vi "GPS通讯(子VI).vi"(8 "error in (no error)":errorcluster caption="错误输入（无错误）") -> ()   [LabVIEW 2016, in "环境动力监测库.lvlib" / "NMEA.lvlib"]
uses:
  NMEA.lvlib
  <vilib>/Plasmionique/MB Master/MB_Master/MB_Master.lvclass
  <vilib>/Plasmionique/MB Master/MB_Master_TCP/MB_Master_TCP.lvclass
  D:/Program Files (x86)/National Instruments/LabVIEW 2016/vi.lib/Plasmionique/MB Master/MB_Master/MB_Master.lvclass
  <vilib>/Instr/_visa.llb/VISA Configure Serial Port (Instr).vi
  <vilib>/Plasmionique/MB Master/MB Master.lvlib
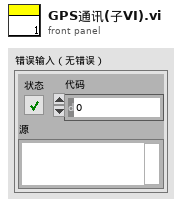
[diagram p1: front panel]
types:
  T1 = cluster{"定位状态":bool, "卫星数量":u16, "时间标识":timestamp, "纬度":dbl, "南北":string, "经度":dbl, "东西":string}
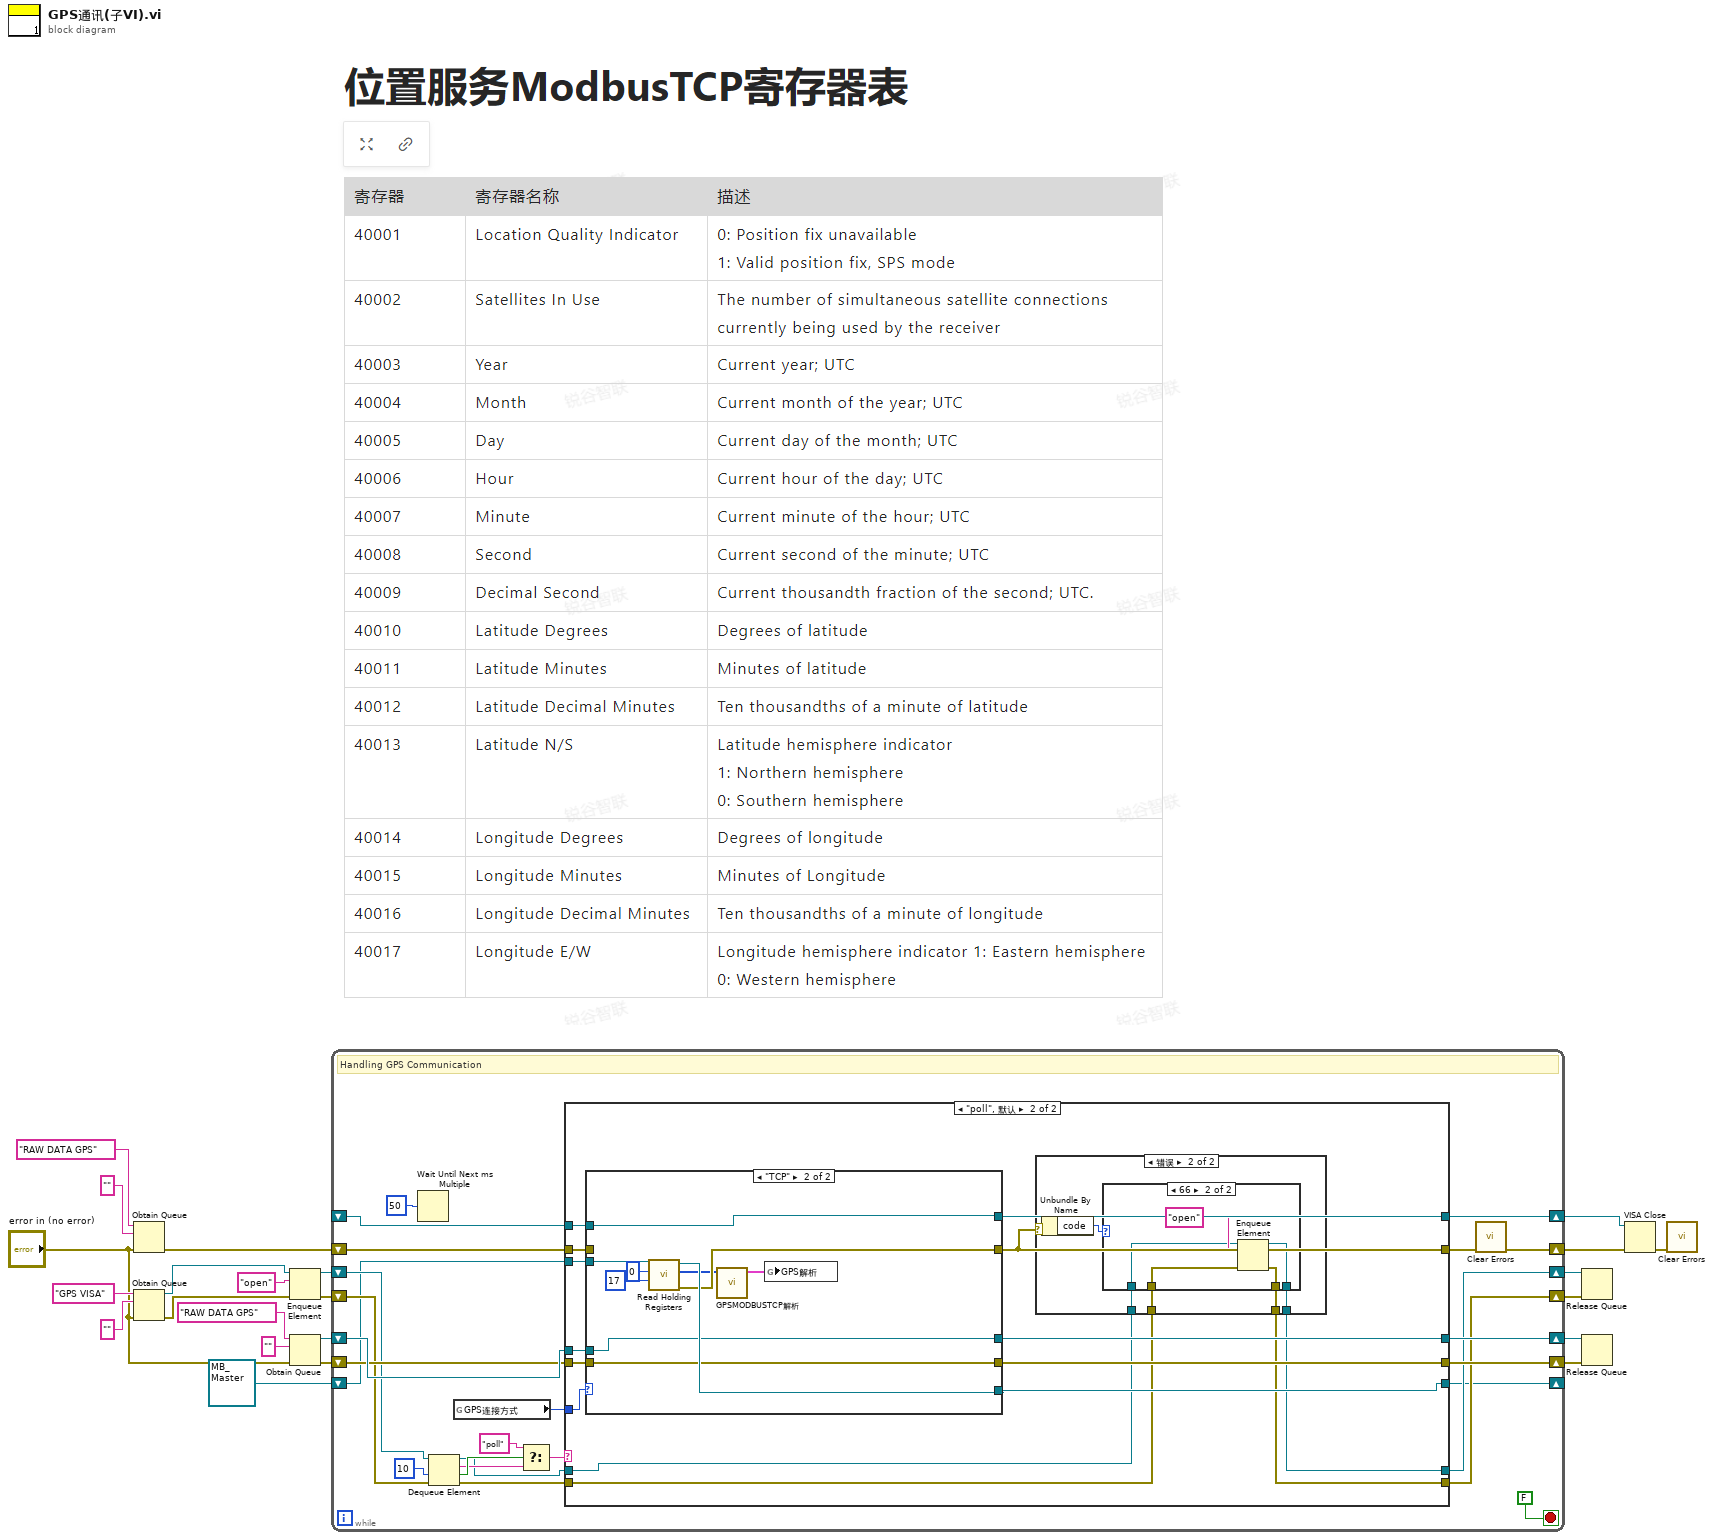
[diagram p0: block diagram]
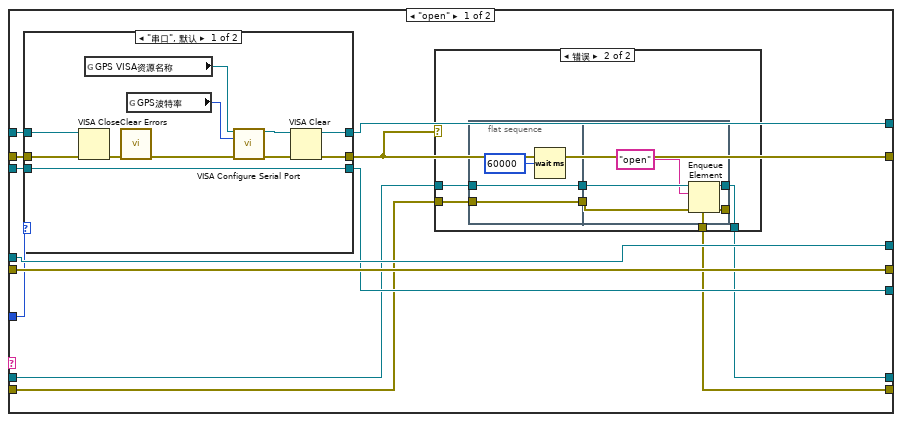
[diagram p2: hidden frame]
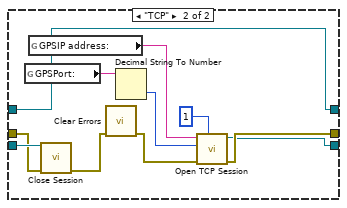
[diagram p4: hidden frame]
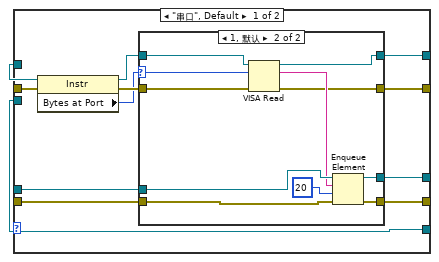
[diagram p7: hidden frame]
diagram:
  n1 = Obtain Queue(name (unnamed)="RAW DATA GPS" ("nom (aucun)"), element data type="" ("expression régulière"), error in (no error)="error in (no error)") -> (error out=w14:errorcluster)  [unwired: 2 in, 2 out]
  n2 = Obtain Queue(name (unnamed)="GPS VISA" ("名称（未命名）"), element data type="" ("名称（未命名）"), error in (no error)="error in (no error)") -> (queue out=w11:refnum<queue>, error out=w10:errorcluster)  [unwired: 2 in, 1 out]
  n3 = Enqueue Element(queue=w11, element="open" ("元素"), error in (no error)=w10) -> (queue out=w8:refnum<queue>, error out=w7:errorcluster)  [unwired: 1 in, 1 out]
  n4 = Obtain Queue(name (unnamed)="RAW DATA GPS" ("nom (aucun)"), element data type="" ("expression régulière"), error in (no error)="error in (no error)") -> (queue out=w4:refnum<queue>, error out=w3:errorcluster)  [unwired: 2 in, 1 out]
  n5 = while {
    shift-right: [w45] -> w18
    shift-left: w3 -> [w47]
    shift-right: [w44] -> w20
    shift-left: _ -> [w43]
    shift-right: [w46] -> w19
    shift-left: w4 -> [w48]
    shift-right: [w39] -> w21
    shift-left: w14 -> [w41]
    shift-right: [w29] -> w22
    shift-left: w7 -> [w37]
    shift-right: [w31] -> w23
    shift-left: w8 -> [w38]
    shift-right: [w25] -> _
    shift-left: refnum<class "MB_Master.lvclass"> refnum ("MB session in") -> [w24]
    stop <- FALSE stop-if-true
    # "Handling GPS Communication"
    n6 = Wait Until Next ms Multiple(millisecond multiple=u32 50 ("attente (ms)")) -> ()  [unwired: 1 out]
    n7 = Dequeue Element(queue=w38, timeout in ms (-1)=10 ("超时毫秒(-1)"), error in (no error)=w37) -> (queue out=w30:refnum<queue>, element=w33:string, timed out?=w35:bool, error out=w28:errorcluster)
    n8 = global read "断电保存全局变量.vi" "GPS连接方式"() -> (w26:enum16{"串口", "TCP"})
    n9 = Select(t="poll" ("名称（未命名）"), s=w35, f=w33) -> (s? t:f=w32:string)
    n10 = case shown="\"poll\", 默认" w32 {
      tunnel: w48 -> [w61 w114]
      tunnel: w47 -> [w60 w113]
      tunnel: [w61 w112] -> w46
      tunnel: [w60 w111] -> w45
      tunnel: [w57 w110] -> w44
      tunnel: w43 -> [w58 w109]
      tunnel: w41 -> [w59 w108]
      tunnel: [w53 w104] -> w40
      tunnel: [w50 w100] -> w31
      tunnel: w30 -> [w52 w103]
      tunnel: [w49 w101] -> w29
      tunnel: w28 -> [w51 w102]
      tunnel: w26 -> [w56 w107]
      tunnel: [w55 w105] -> w25
      tunnel: w24 -> [w54 w106]
      frame "open" {
        n11 = case shown="\"串口\", 默认" w56 {
          tunnel: w59 -> [w85 w91]
          tunnel: w58 -> [w84 w99]
          tunnel: [w81 w99] -> w57
          tunnel: [w79 w93] -> w53
          tunnel: [w78 w89] -> w55
          tunnel: w54 -> [w78 w92]
          frame "串口", Default {
            n12 = VISA Close(VISA resource name=w84, error in (no error)=w85) -> (error out=w83:errorcluster)
            n13 = global read "断电保存全局变量.vi" "GPS VISA资源名称"() -> (w87:refnum<visa-resource-name>)
            n14 = call <vilib>:"Clear Errors.vi"("error in (no error)"=w83) -> ("error out"=w82:errorcluster)  [unwired: 5 in, 1 out]
            n15 = global read "断电保存全局变量.vi" "GPS波特率"() -> (w88:u32)
            n16 = call-poly "VISA Configure Serial Port"("VISA resource name"=w87, "baud rate (9600)"=w88, "error in (no error)"=w82) -> ("VISA resource name out"=w86:refnum<visa-resource-name>, "error out"=w80:errorcluster)  [unwired: 11 in]
            n17 = VISA Clear(VISA resource name=w86, error in (no error)=w80) -> (VISA resource name out=w81:refnum<visa-resource-name>, error out=w79:errorcluster)
          }
          frame "TCP" {
            n18 = global read "断电保存全局变量.vi" "GPSPort:"() -> (w96:string)
            n19 = global read "断电保存全局变量.vi" "GPSIP address:"() -> (w97:string)
            n20 = call-dynamic "Close Session.vi"("error in (no error)"=w91, "MB session in"=w92) -> ("error out"=w90:errorcluster)  [unwired: 9 in]
            n21 = call <vilib>:"Clear Errors.vi"("error in (no error)"=w90) -> ("error out"=w94:errorcluster)  [unwired: 5 in, 1 out]
            n22 = Decimal String To Number(string=w96) -> (number=w95:i32)  [unwired: 2 in, 1 out]
            n23 = call <vilib>:"Open TCP Session.vi"("Slave ID (255)"=u8 1, "error in (no error)"=w94, "Port (502)"=w95, "IP Address"=w97) -> ("error out"=w93:errorcluster, "MB_TCP session"=w89:refnum<class "MB_Master_TCP.lvclass">)  [unwired: 6 in]
          }
        }
        n24 = case shown="错误" w53 {
          tunnel: w52 -> [w63 w69]
          tunnel: w51 -> [w62 w68]
          tunnel: [w63 w67] -> w50
          tunnel: [w62 w66] -> w49
          frame No Error {
          }
          frame Error {
            n25 = flat-sequence {
              tunnel: w68 -> [w71]
              tunnel: w69 -> [w72]
              tunnel: [w72] -> w65
              tunnel: [w71] -> w64
              tunnel: [w74] -> w67
              tunnel: [w73] -> w66
              tunnel: w65 -> [w77]
              tunnel: w64 -> [w76]
              frame #0 {
                n26 = Wait (ms)(milliseconds to wait=u32 60000 ("等待时间（毫秒）")) -> ()  [unwired: 1 out]
              }
              frame #1 {
                n27 = Enqueue Element(queue=w77, element="open" ("名称（未命名）"), error in (no error)=w76) -> (queue out=w74:refnum<queue>, error out=w73:errorcluster)  [unwired: 1 in, 1 out]
              }
            }
          }
        }
      }
      frame "poll", Default {
        n28 = case shown="\"TCP\"" w107 {
          tunnel: w114 -> [w141 w160]
          tunnel: w113 -> [w140 w159]
          tunnel: [w139 w160] -> w112
          tunnel: [w138 w159] -> w111
          tunnel: [w137 w166] -> w110
          tunnel: w109 -> [w136 w166]
          tunnel: w108 -> [w135 _]
          tunnel: [w134 w161] -> w104
          tunnel: w106 -> [w130 w165]
          tunnel: [w130 w162] -> w105
          frame "串口", Default {
            n29 = property class="Instr"(reference=w136, error in=w135) -> (reference out=w133:refnum<visa-resource-name>, error out=w132:errorcluster, "Bytes at Port"=w131:u32)
            n30 = case shown="1, 默认" w131 {
              selector: w131 -> [_ w147]
              tunnel: w141 -> [w142 w156]
              tunnel: w140 -> [w143 w155]
              tunnel: [w142 w154] -> w139
              tunnel: [w143 w153] -> w138
              tunnel: [w144 w151] -> w137
              tunnel: w133 -> [w144 w150]
              tunnel: w132 -> [w145 w149]
              tunnel: [w145 w148] -> w134
              frame 0 {
              }
              frame 1, Default {
                n31 = VISA Read(VISA resource name=w150, byte count=w147, error in (no error)=w149) -> (VISA resource name out=w151:refnum<visa-resource-name>, read buffer=w152:string, error out=w148:errorcluster)  [unwired: 1 out]
                n32 = Enqueue Element(queue=w156, element=w152, timeout in ms (-1)=20 ("timeout en ms (-1)"), error in (no error)=w155) -> (queue out=w154:refnum<queue>, error out=w153:errorcluster)  [unwired: 1 out]
              }
            }
          }
          frame "TCP" {
            n33 = call <vilib>:"Read Holding Registers.vi"("quantity"=u16 17, "starting address"=u16 0, "MB session in"=w165) -> ("error out"=w161:errorcluster, "Registers"=w158:u16[], "MB session out"=w162:refnum<class "MB_Master.lvclass">)  [unwired: 6 in]
            n34 = call "GPSMODBUSTCP解析.vi"("Registers"=w158) -> ("GPS解析"=w157:T1)  [unwired: 10 in]
            n35 = global write "NMEA过程全局变量.vi" "GPS解析"(w157) -> ()
          }
        }
        n36 = case shown="错误" w104 {
          selector: w104 -> [_ w122]
          tunnel: w103 -> [w116 w120]
          tunnel: w102 -> [w115 w119]
          tunnel: [w115 w118] -> w101
          tunnel: [w116 w117] -> w100
          frame No Error {
          }
          frame Error {
            n37 = Unbundle By Name(w122) -> ("code"=w121:i32)
            n38 = case shown="66" w121 {
              tunnel: w120 -> [w123 w128]
              tunnel: w119 -> [w124 w127]
              tunnel: [w124 w126] -> w118
              tunnel: [w123 w125] -> w117
              frame 0, Default {
              }
              frame 66 {
                n39 = Enqueue Element(queue=w128, element="open" ("名称（未命名）"), error in (no error)=w127) -> (queue out=w125:refnum<queue>, error out=w126:errorcluster)  [unwired: 1 in, 1 out]
              }
            }
          }
        }
      }
    }
    n40 = call <vilib>:"Clear Errors.vi"("error in (no error)"=w40) -> ("error out"=w39:errorcluster)  [unwired: 5 in, 1 out]
  }
  n41 = Release Queue(queue=w23, error in (no error)=w22) -> ()  [unwired: 1 in, 3 out]
  n42 = Release Queue(queue=w19, error in (no error)=w18) -> ()  [unwired: 1 in, 3 out]
  n43 = VISA Close(VISA resource name=w20, error in (no error)=w21) -> (error out=w17:errorcluster)
  n44 = call <vilib>:"Clear Errors.vi"("error in (no error)"=w17) -> ()  [unwired: 5 in, 2 out]
